vi "SSC DCPower Configure Measurements.vi"(0 "DCPower SSC in":T2[](array[typedef]), 5 "Measurement Mode":T1 caption="Measurement Mode (Auto)", 11 "error in":errorcluster) -> (4 "DCPower SSC out":T2[](array[typedef]), 15 "error out":errorcluster)   [LabVIEW 2020]
doc: "This VI configures the measurement mode for the sessions.\n\nThe (Auto) setting automatically chooses the optimal measurement mode individually for the instrument model in each session.\n\nFrom a test time perspective Software Triggered measurements are better than using Measure Multiple, but Software Triggering isn't supported by all devices, and enabling them can make debugging in the Digital Pattern Editor more difficult.\n\nMeasure Multiple works for all devices and allows for easier debugging, but it takes longer to fetch measurements than the Software Triggered method."
uses:
  SSC DCPower.ctl
  Measure/SSC DCPower Measurement Mode.ctl
  Measure/SSC DCPower Debug Global.vi
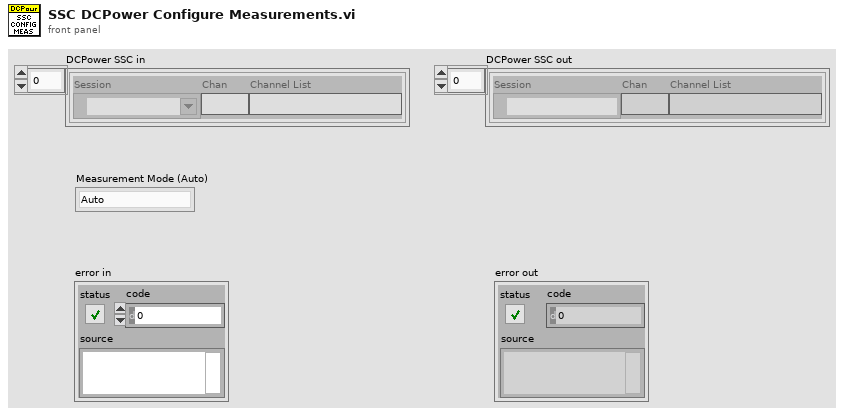
[diagram p1: front panel]
types:
  T1 = typedef "SSC DCPower Measurement Mode.ctl" = enum16{"Auto", "Measure Multiple", "Software Triggers"}
  T2 = typedef "SSC DCPower.ctl" = cluster{"Session":refnum<k15>, "Chan":string, "Channel List":string}
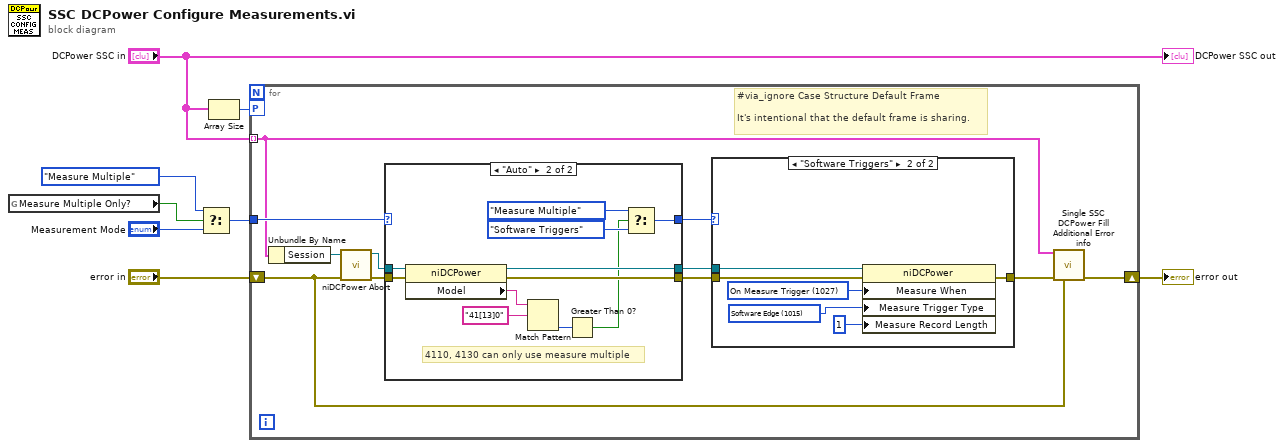
[diagram p0: block diagram]
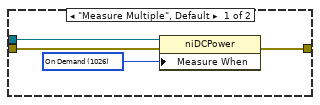
[diagram p3: hidden frame]
diagram:
  n1 = global read "SSC DCPower Debug Global.vi" "Measure Multiple Only?"() -> (w2:bool)
  n2 = Select(t=SSC_DCPower_Measurement_Mode."Measure Multiple", s=w2, f="Measurement Mode") -> (s? t:f=w5:T1)
  n3 = Array Size(array="DCPower SSC in") -> (size(s)=w3:i32)
  n4 = for {
    tunnel: w5 -> [w17]
    shift-right: [w11] -> w7
    shift-left: "error in" -> [w9]
    tunnel: "DCPower SSC in" -> [w10] mode=indexing
    workers-P: w3 -> [_]
    # "#via_ignore Case Structure Default Frame\n\nIt's intentional that the default frame is sharing."
    n5 = Unbundle By Name(w10) -> ("Session"=w13:refnum<k15>)
    n6 = call <instrlib>:"niDCPower Abort.vi"("error in (no error)"=w9, "instrument handle"=w13) -> ("error out"=w14:errorcluster, "instrument handle out"=w12:refnum<k15>)  [unwired: 8 in]
    n7 = case shown="\"Auto\"" w17 {
      selector: w17 -> [w20 _]
      tunnel: w14 -> [w22 w33]
      tunnel: [w22 w32] -> w18
      tunnel: w12 -> [w21 w31]
      tunnel: [w21 w30] -> w16
      tunnel: [w20 w28] -> w15
      frame Default {
      }
      frame "Auto" {
        # "4110, 4130 can only use measure multiple"
        n8 = property class="niDCPower"(reference=w31, error in=w33) -> (reference out=w30:refnum<k15>, error out=w32:errorcluster, "Model"=w25:string)
        n9 = Match Pattern(string=w25, regular expression="41[13]0") -> (offset past match=w24:i32)  [unwired: 1 in, 3 out]
        n10 = Greater Than 0?(x=w24) -> (x > 0?=w23:bool)
        n11 = Select(t=SSC_DCPower_Measurement_Mode."Measure Multiple" ("Measurment Mode 2"), s=w23, f=SSC_DCPower_Measurement_Mode."Software Triggers" ("Measurment Mode 2")) -> (s? t:f=w28:T1)
      }
    }
    n12 = case shown="\"Software Triggers\"" w15 {
      tunnel: w18 -> [w37 w43]
      tunnel: [w36 w42] -> w19
      tunnel: w16 -> [w34 w38]
      frame "Measure Multiple", Default {
        w35 = 1026 items=["Automatically after Source Complete"=1025, "On Demand"=1026, "On Measure Trigger"=1027] ("Measurement:Advanced:Measure When")
        n13 = property class="niDCPower"(reference=w34, error in=w37, "Measure When"=w35) -> (error out=w36:errorcluster)  [unwired: 1 out]
      }
      frame "Software Triggers" {
        w40 = 1015 items=["Digital Edge"=1014, "Software Edge"=1015, "None"=1012] ("Triggers:Measure Trigger:Trigger Type")
        w41 = 1027 items=["Automatically after Source Complete"=1025, "On Demand"=1026, "On Measure Trigger"=1027] ("Measurement:Advanced:Measure When")
        n14 = property class="niDCPower"(reference=w38, error in=w43, "Measure When"=w41, "Measure Trigger Type"=w40, "Measure Record Length"=1 ("Measurement:Measure Record Length")) -> (error out=w42:errorcluster)  [unwired: 1 out]
      }
    }
    n15 = call "Single SSC DCPower Fill Additional Error info.vi"("DCPower SSC in"=w10, "error in"=w19, "previous error in"=w9) -> ("error out"=w11:errorcluster)  [unwired: 12 in]
  }
  "error out" <- w7
  "DCPower SSC out" <- "DCPower SSC in"
